vi "Flatten.vi"(8 "error in":errorcluster, 9 "Data":T1) -> (0 "error out":errorcluster, 2 "Buffer":u8[](array[numeric]) format="%.0x")   [LabVIEW 2020, in "TcpClientList.lvlib"]
uses:
  TcpClientList.lvlib
  Data.ctl
  TcpClientInfo/TcpClientInfo.lvlib
  TcpClientInfo/Data.ctl
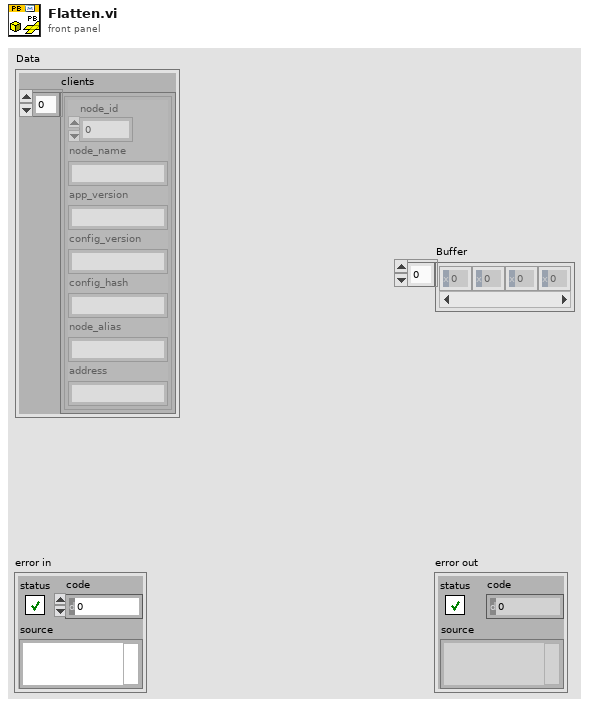
[diagram p1: front panel]
types:
  T1 = typedef "TcpClientList.lvlib/Data.ctl" = cluster{"clients":T2[]}
  T2 = typedef "TcpClientInfo.lvlib/Data.ctl" = cluster{"node_id":u32, "node_name":string, "app_version":string, "config_version":string, "config_hash":string, "node_alias":string, "address":string}
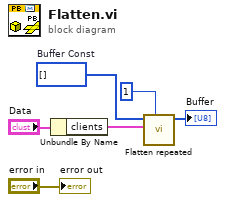
[diagram p0: block diagram]
diagram:
  w4 = u8[] []  # Buffer Const
  n1 = Unbundle By Name("Data") -> ("clients"=w3:T2[])
  n2 = call "Flatten repeated.vi"("Field Number"=1, "Data"=w3, "Buffer in"=w4) -> ("Buffer"=→"Buffer":u8[])  [unwired: 8 in]
  "error out" <- "error in"
